vi "VIS-IR_WRITE_L.vi"(6 "val":u32, 8 "error in (no error)":errorcluster, 9 "offset":u32, 10 "drv":u32=1, 11 "VIS-IR in":refnum<class "VIS-NIR.lvclass">) -> (0 "error out":errorcluster, 3 "VIS-IR out":refnum<class "VIS-NIR.lvclass">)   [LabVIEW 2015, in "VIS-NIR.lvclass"]
uses:
  VIS-NIR.lvclass
  Detector.lvclass/Detector.ctl
  Detector.lvclass
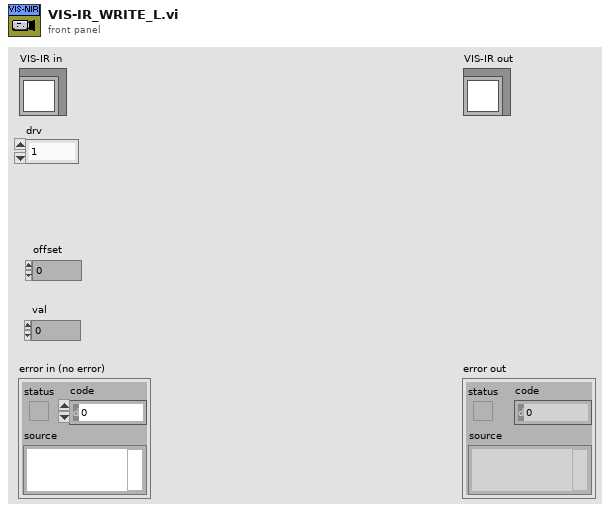
[diagram p1: front panel]
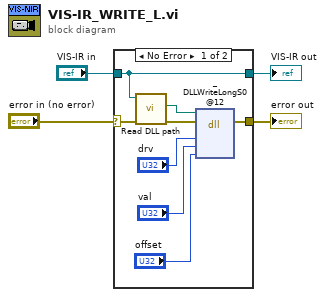
[diagram p0: block diagram]
diagram:
  n1 = case shown="No Error" "error in (no error)" {
    selector: "error in (no error)" -> [w11 w14]
    tunnel: [w5 w14] -> w3
    tunnel: [w12 w13] -> w1
    tunnel: "VIS-IR in" -> [w12 w13]
    frame No Error {
      n2 = call "Read DLL path.vi"("error in (no error)"=w11, "Detector in"=w12) -> ("error out"=w6:errorcluster, "DLL path"=w7:path)  [unwired: 7 in, 1 out]
      n3 = dll-call lib="G:/SD/TRANCON/DLL/ESLSCDLL.dll" fn="_DLLWriteLongS0@12" ("lwlscdll.dll:DLLWriteLongS0")(path in=w7, error in=w6, "drv"="drv", "DataByte"="val", "PortOff"="offset") -> (error out=w5:errorcluster)  [unwired: 5 in, 1 out]
    }
    frame Error {
    }
  }
  "error out" <- w3
  "VIS-IR out" <- w1
